vi "Set Optimiser Strategy.vi"(8 "error in (no error)":errorcluster, 9 "Value":dbl, 10 "Optimisation method":T1, 11 "Optimiser SBlock in":refnum<class "Optimiser SBlock.lvclass">) -> (0 "error out":errorcluster, 3 "Optimiser SBlock out":refnum<class "Optimiser SBlock.lvclass">)   [LabVIEW 2020, in "TALOS.lvlib" / "Run Utilities.lvlib" / "Optimiser SBlock.lvclass"]
uses:
  Optimiser SBlock.lvclass
  Optimiser Cell/Optimisation Strategy.ctl
  Optimiser Cell/Optimiser Cell.lvclass
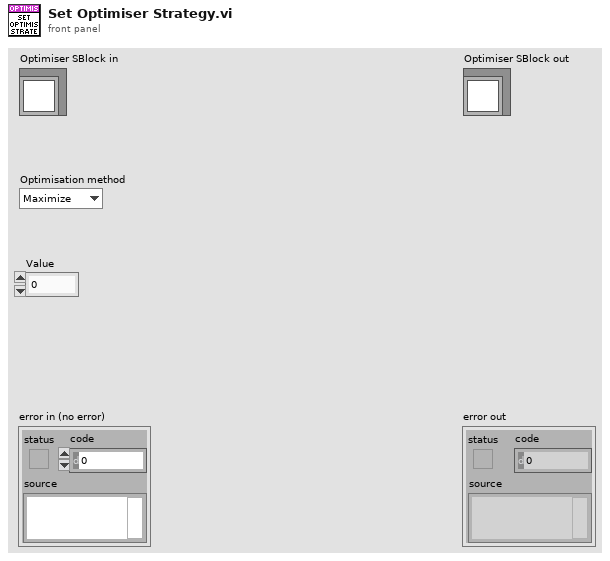
[diagram p1: front panel]
types:
  T1 = typedef "TALOS.lvlib/Run Utilities.lvlib/Optimiser Cell.lvclass/Optimisation Strategy.ctl" = enum16{"Maximize", "Minimize", "Value"}
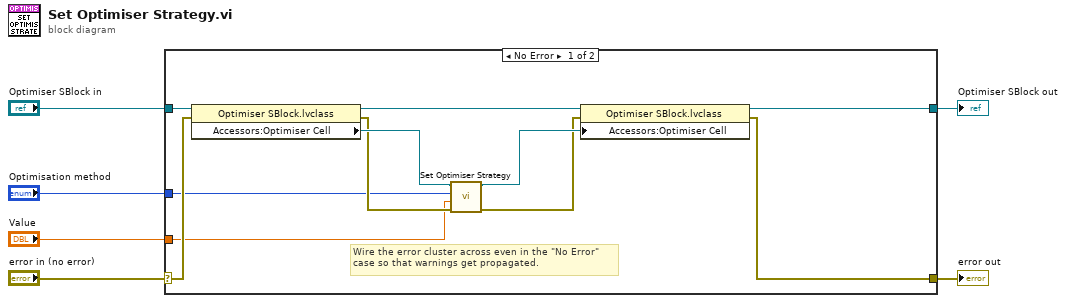
[diagram p0: block diagram]
diagram:
  n1 = case shown="No Error" "error in (no error)" {
    selector: "error in (no error)" -> [w13 w19]
    tunnel: [w14 w19] -> w5
    tunnel: [w15 w18] -> w3
    tunnel: "Optimiser SBlock in" -> [w17 w18]
    tunnel: "Optimisation method" -> [w8 _]
    tunnel: "Value" -> [w7 _]
    frame No Error {
      # "Wire the error cluster across even in the \"No Error\"\ncase so that warnings get propagated."
      n2 = property class="Optimiser SBlock.lvclass"(reference=w17, error in=w13) -> (reference out=w16:refnum<class "Optimiser SBlock.lvclass">, error out=w9:errorcluster, "Accessors:Optimiser Cell"=w12:refnum<class "Optimiser Cell.lvclass">)
      n3 = call-dynamic "Set Optimiser Strategy.vi"("error in (no error)"=w9, "Value"=w7, "Optimisation method"=w8, "Optimiser Cell in"=w12) -> ("error out"=w10:errorcluster, "Optimiser Cell out"=w11:refnum<class "Optimiser Cell.lvclass">)  [unwired: 6 in]
      n4 = property class="Optimiser SBlock.lvclass"(reference=w16, error in=w10, "Accessors:Optimiser Cell"=w11) -> (reference out=w15:refnum<class "Optimiser SBlock.lvclass">, error out=w14:errorcluster)
    }
    frame Error {
    }
  }
  "error out" <- w5
  "Optimiser SBlock out" <- w3
